vi "readPIDSetting.vi"(8 "Error In":errorcluster) -> (0 "Error Out":errorcluster, 1 "Ch3 PID out":T1, 2 "Ch2 PID out":T1, 3 "Ch1 PID out":T1)   [LabVIEW 2020]
uses:
  <vilib>/Utility/config.llb/Read Key (Double).vi
  <vilib>/Utility/config.llb/NI_LVConfig.lvlib
panel:
  out "Ch4 PID out":T1
  out "Setting file path":path
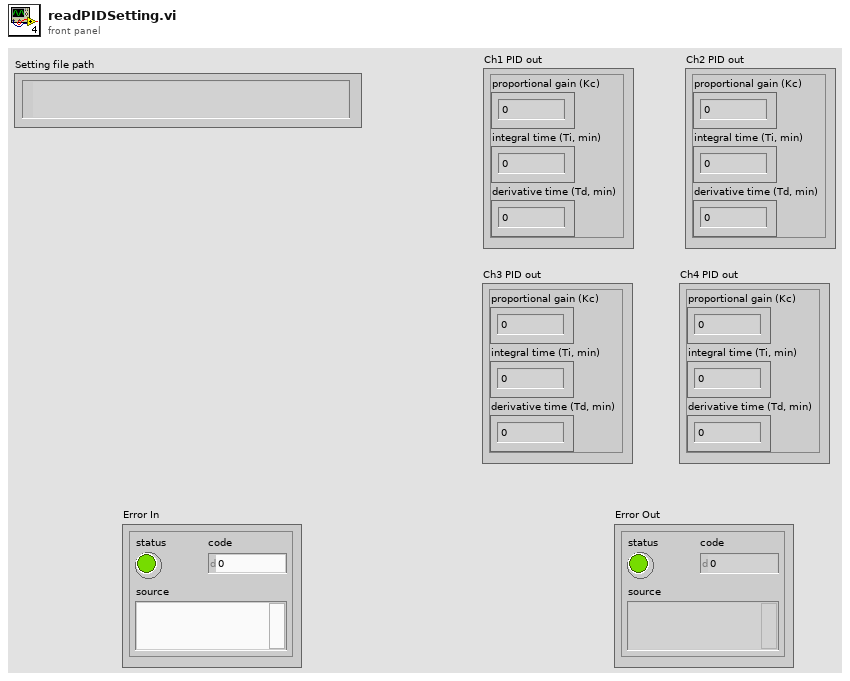
[diagram p1: front panel]
types:
  T1 = cluster{"proportional gain (Kc)":dbl, "integral time (Ti, min)":dbl, "derivative time (Td, min)":dbl}
  T2 = typedef "NI_LVConfig.lvlib/Config Data RefNum.ctl" = refnum<k1>
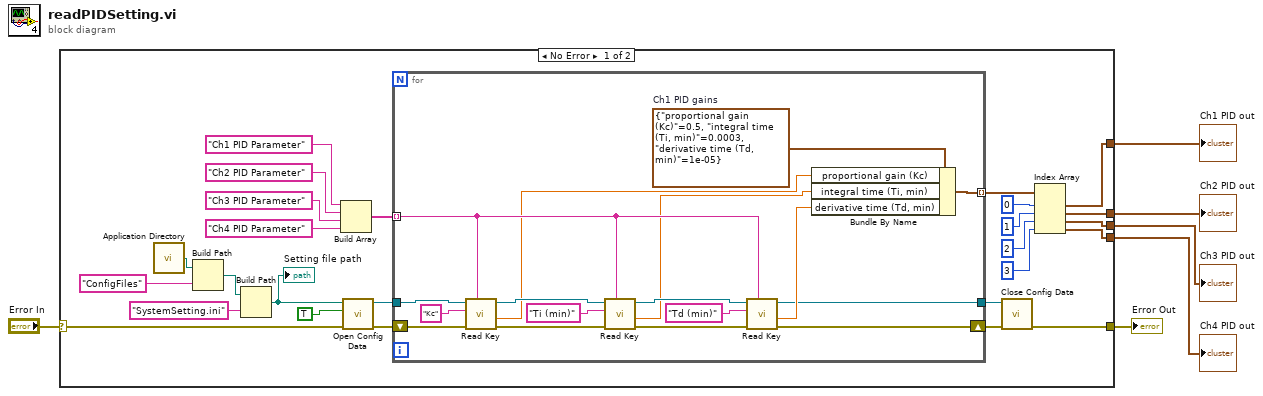
[diagram p0: block diagram]
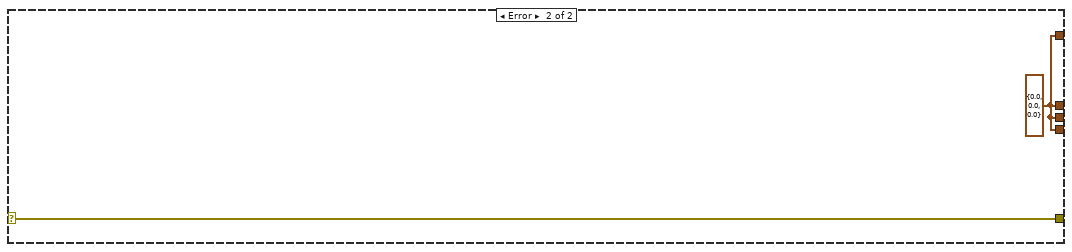
[diagram p2: hidden frame]
diagram:
  n1 = case shown="No Error" "Error In" {
    selector: "Error In" -> [w26 w51]
    tunnel: [w17 w51] -> w5
    tunnel: [w14 w50] -> w4
    tunnel: [w11 w50] -> w3
    tunnel: [w10 w50] -> w2
    tunnel: [w7 w50] -> w1
    frame No Error {
      n2 = call <vilib>:"Application Directory.vi"() -> ("Application Directory"=w32:path)
      n3 = Build Path(base path=w32, name or relative path="ConfigFiles") -> (appended path=w30:path)
      n4 = Build Path(base path=w30, name or relative path="SystemSetting.ini") -> (appended path=w27:path)
      "Setting file path" <- w27
      n5 = Build Array("Ch1 PID Parameter", "Ch2 PID Parameter", "Ch3 PID Parameter", "Ch4 PID Parameter") -> (w22:string[])
      n6 = call <vilib>:"Open Config Data.vi"("error in (no error)"=w26, "create file if necessary (T)"=TRUE, "configuration file path"=w27) -> ("error out"=w21:errorcluster, "refnum"=w20:T2)  [unwired: 6 in, 1 out]
      n7 = for {
        tunnel: w22 -> [w40] mode=indexing
        tunnel: w20 -> [w48]
        shift-right: [w34] -> w18
        shift-left: w21 -> [w49]
        tunnel: [w35] -> w16 mode=indexing
        tunnel: [w33] -> w19
        w39 = T1 {"proportional gain (Kc)"=0.5, "integral time (Ti, min)"=0.0003, "derivative time (Td, min)"=1e-05}  # Ch1 PID gains
        n8 = call-poly <vilib>:"Read Key.vi"("section"=w40, "error in (no error)"=w49, "key"="Kc", "refnum"=w48) -> ("error out"=w45:errorcluster, "value"=w38:dbl, "refnum out"=w46:T2)  [unwired: 4 in, 1 out]
        n9 = call-poly <vilib>:"Read Key.vi"("section"=w40, "error in (no error)"=w45, "key"="Ti (min)", "refnum"=w46) -> ("error out"=w42:errorcluster, "value"=w37:dbl, "refnum out"=w43:T2)  [unwired: 4 in, 1 out]
        n10 = call-poly <vilib>:"Read Key.vi"("section"=w40, "error in (no error)"=w42, "key"="Td (min)", "refnum"=w43) -> ("error out"=w34:errorcluster, "value"=w36:dbl, "refnum out"=w33:T2)  [unwired: 4 in, 1 out]
        n11 = Bundle By Name(cluster=w39, "proportional gain (Kc)"=w38, "integral time (Ti, min)"=w37, "derivative time (Td, min)"=w36) -> (w35:T1)
      }
      n12 = call <vilib>:"Close Config Data.vi"("error in (no error)"=w18, "refnum"=w19) -> ("error out"=w17:errorcluster)  [unwired: 8 in, 1 out]
      n13 = Index Array(array=w16, index #1=0 ("index"), index #2=1 ("index"), index #3=2 ("index"), index #4=3 ("index")) -> (element #1=w14:T1, element #2=w11:T1, element #3=w10:T1, element #4=w7:T1)
    }
    frame Error {
      w50 = T1 {"proportional gain (Kc)"=0.0, "integral time (Ti, min)"=0.0, "derivative time (Td, min)"=0.0} ("Ch1 PID gains")
    }
  }
  "Error Out" <- w5
  "Ch1 PID out" <- w4
  "Ch2 PID out" <- w3
  "Ch3 PID out" <- w2
  "Ch4 PID out" <- w1
